vi "Configure IO Port.vi"(5 "Bit 4 Polarity (0: High)":u16(ring) items=["High", "Low"], 6 "Auto Clear Delay (1.0 s)":dbl=1.0, 7 "Bit 4 Operation (0: End of Test)":u16(ring) items=["End of Test", "Busy"], 8 "error in (no error)":errorcluster, 9 "Enable Auto Clear (T:Enable)":bool=TRUE, 10 "Operating Mode (0: 3-bit)":u16(ring) items=["3-bit", "4-bit"], 11 "VISA resource name":refnum<visa-resource-name>) -> (0 "error out":errorcluster, 3 "VISA resource name out":refnum<visa-resource-name>)   [LabVIEW 2017, in "Keithley 24XX.lvlib"]
doc: "Configures I/O port behavior during limit testing. Settings include configuration of signaling bit behavior and auto-clearing of output patterns."
uses:
  Keithley 24XX.lvlib
panel:
  # "Bit 4 Behavior (3-bit mode only)"
  # "Auto Clear Settings"
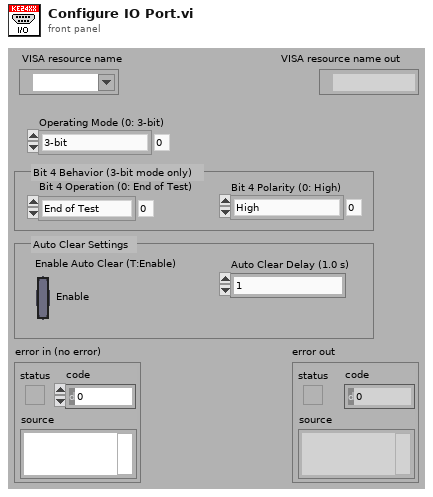
[diagram p1: front panel]
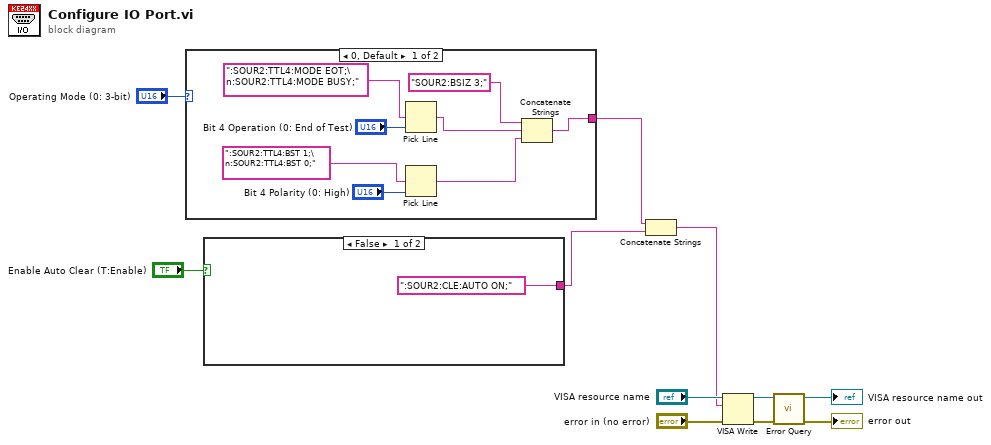
[diagram p0: block diagram]
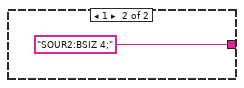
[diagram p2: hidden frame]
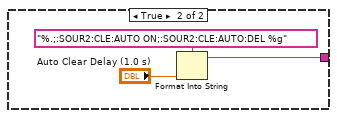
[diagram p3: hidden frame]
diagram:
  n1 = case shown="0, Default" "Operating Mode (0: 3-bit)" {
    tunnel: [w12 "SOUR2:BSIZ 4;"] -> w3
    frame 0, Default {
      n2 = Pick Line(multi-line string=":SOUR2:TTL4:MODE EOT;\n:SOUR2:TTL4:MODE BUSY;", line index="Bit 4 Operation (0: End of Test)") -> (output string=w14:string)  [unwired: 1 in]
      n3 = Pick Line(multi-line string=":SOUR2:TTL4:BST 1;\n:SOUR2:TTL4:BST 0;", line index="Bit 4 Polarity (0: High)") -> (output string=w13:string)  [unwired: 1 in]
      n4 = Concatenate Strings("SOUR2:BSIZ 3;", w14, w13) -> (w12:string)
    }
    frame 1 {
    }
  }
  n5 = case shown="False" "Enable Auto Clear (T:Enable)" {
    tunnel: [":SOUR2:CLE:AUTO ON;" w22] -> w1
    frame False {
    }
    frame True {
      n6 = Format Into String(format string="%.;:SOUR2:CLE:AUTO ON;:SOUR2:CLE:AUTO:DEL %g", "Auto Clear Delay (1.0 s)") -> (resulting string=w22:string)  [unwired: 2 in, 1 out]
    }
  }
  n7 = Concatenate Strings(w3, w1) -> (w2:string)
  n8 = VISA Write(VISA resource name="VISA resource name", write buffer=w2, error in (no error)="error in (no error)") -> (VISA resource name out=w7:refnum<visa-resource-name>, error out=w6:errorcluster)  [unwired: 1 out]
  n9 = call "Error Query.vi"("error in (no error)"=w6, "VISA resource name"=w7) -> ("error out"=→"error out":errorcluster, "VISA resource name out"=→"VISA resource name out":refnum<visa-resource-name>)  [unwired: 6 in, 2 out]
